vi "Next Step.vi"(8 "error in (no error)":errorcluster, 11 "Wavelength Digikröm in":refnum<class "Wavelength Digikröm.lvclass">) -> (0 "error out":errorcluster, 1 "Current Step":u32, 2 "Current Position":dbl, 3 "Wavelength Digikröm out":refnum<class "Wavelength Digikröm.lvclass">)   [LabVIEW 2015, in "Wavelength Digikröm.lvclass"]
uses:
  Scanner/Scanner.lvclass
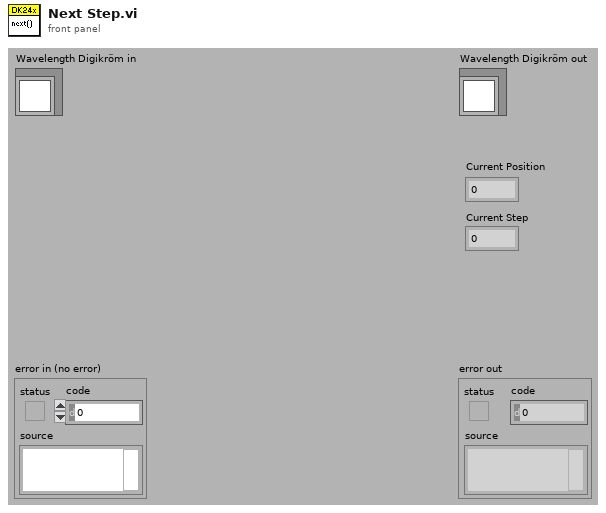
[diagram p1: front panel]
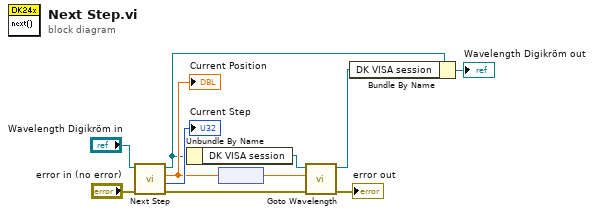
[diagram p0: block diagram]
diagram:
  n1 = call-parent "Next Step.vi"("error in (no error)"="error in (no error)", "Scanner in"="Wavelength Digikröm in") -> ("error out"=w5:errorcluster, "Current Step"=→"Current Step":u32, "Current Position"=w2:dbl, "Scanner out"=w1:refnum<class "Wavelength Digikröm.lvclass">)  [unwired: 6 out]
  "Current Position" <- w2
  n2 = Unbundle By Name(w1) -> ("DK VISA session"=w8:refnum<visa-resource-name>)
  n3 = node(w2) -> (w6:dbl[unit])
  n4 = call "Goto Wavelength.vi"("error in (no error)"=w5, "WAVELENGTH"=w6, "VISA resource name"=w8) -> ("error out"=→"error out":errorcluster, "VISA resource name out"=w7:refnum<visa-resource-name>)  [unwired: 7 out]
  n5 = Bundle By Name(cluster=w1, "DK VISA session"=w7) -> (→"Wavelength Digikröm out":refnum<class "Wavelength Digikröm.lvclass">)
